vi "Configure PRACH Trigger.vi"(5 "Minimum Trigger Gap (50e-6)":dbl=5e-05 format="%^.3e", 6 "Trigger Threshold (-20)":i32=-20, 7 "Trigger Slope (Rising edge)":i32(ring) items=["Rising edge", "Falling edge"], 8 "error in (no error)":errorcluster, 9 "Trigger Source (\"IF Power\")":string="IF Power", 10 "Instance (1)":T1=1, 11 "VISA resource name":refnum<visa-resource-name>) -> (0 "error out":errorcluster, 3 "VISA resource name out":refnum<visa-resource-name>)   [LabVIEW 2020, in "Rohde&Schwarz CMWXP NR FR1 Measurement.lvlib"]
doc: "Configures multi evaluation measurement trigger subsystem.\n\nAttributes:\nRSCMWXPNRFR1M_ATTR_PRACH_TRIGGER_SOURCE\nRSCMWXPNRFR1M_ATTR_PRACH_TRIGGER_SLOPE\nRSCMWXPNRFR1M_ATTR_PRACH_TRIGGER_THRESHOLD\nRSCMWXPNRFR1M_ATTR_PRACH_MINIMUM_TRIGGER_GAP\n\nRemote-control commands:\nTRIGger:NRSub:MEAS<i>:PRACh:SOURce\nTRIGger:NRSub:MEAS<i>:PRACh:SLOPe\nTRIGger:NRSub:MEAS<i>:PRACh:THReshold\nTRIGger:NRSub:MEAS<i>:PRACh:MGAP"
uses:
  <instrlib>/Rohde&Schwarz CMWXP NR FR1 Measurement/Rohde&Schwarz CMWXP NR FR1 Measurement.lvlib
  <instrlib>/Rohde&Schwarz CMWXP NR FR1 Measurement/Private/_Instance.ctl
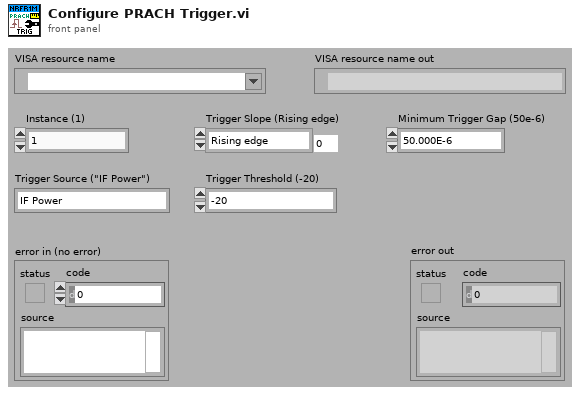
[diagram p1: front panel]
types:
  T1 = typedef "Rohde&Schwarz CMWXP NR FR1 Measurement.lvlib/_Instance.ctl" = i32
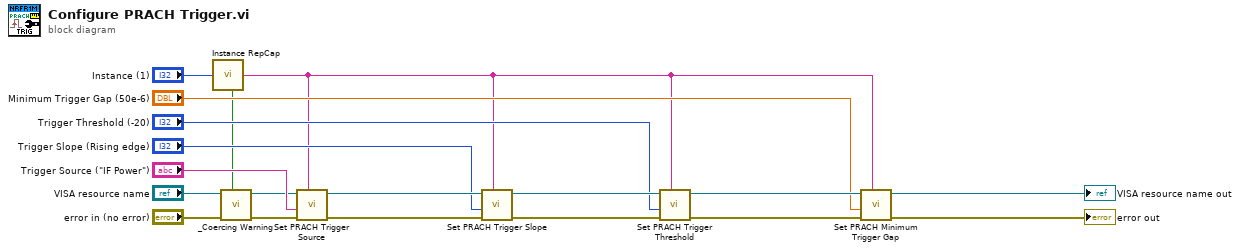
[diagram p0: block diagram]
diagram:
  n1 = call <instrlib>:"Instance RepCap.vi"("Instance In"="Instance (1)") -> ("In Range?"=w2:bool, "RepCap Identifier Out"=w1:string)  [unwired: 1 in]
  n2 = call <instrlib>:"_Coercing Warning.vi"("In Range?"=w2, "error in (no error)"="error in (no error)", "VISA resource name"="VISA resource name") -> ("error out"=w5:errorcluster, "VISA resource name out"=w4:refnum<visa-resource-name>)  [unwired: 7 in]
  n3 = call "Set PRACH Trigger Source"("Repeated Capabilities"=w1, "error in (no error)"=w5, "PRACH Trigger Source ()"="Trigger Source (\"IF Power\")", "instrument handle"=w4) -> ("error out"=w17:errorcluster, "instrument handle out"=w18:refnum<visa-resource-name>)  [unwired: 6 in]
  n4 = call "Set PRACH Trigger Slope"("Repeated Capabilities"=w1, "error in (no error)"=w17, "PRACH Trigger Slope (0 - Rising edge)"="Trigger Slope (Rising edge)", "instrument handle"=w18) -> ("error out"=w14:errorcluster, "instrument handle out"=w15:refnum<visa-resource-name>)  [unwired: 6 in]
  n5 = call "Set PRACH Trigger Threshold"("Repeated Capabilities"=w1, "error in (no error)"=w14, "PRACH Trigger Threshold (0)"="Trigger Threshold (-20)", "instrument handle"=w15) -> ("error out"=w9:errorcluster, "instrument handle out"=w10:refnum<visa-resource-name>)  [unwired: 6 in]
  n6 = call "Set PRACH Minimum Trigger Gap"("Repeated Capabilities"=w1, "error in (no error)"=w9, "PRACH Minimum Trigger Gap (0.0)"="Minimum Trigger Gap (50e-6)", "instrument handle"=w10) -> ("error out"=→"error out":errorcluster, "instrument handle out"=→"VISA resource name out":refnum<visa-resource-name>)  [unwired: 6 in]
